vi "TXSIG_Generate(SubVi).vi"(5 "Chip_rate_Threshold":dbl=5.0 format="%#_13g", 7 "ThresHold":dbl=5.0 format="%#_13g", 9 "Rc":dbl=5500.0 format="%#_13g", 10 "길이":i32=256, 11 "이름 또는 상대 경로":string) -> (1 "TXN":dbl[](array[numeric]), 2 "TXP":dbl[](array[numeric]), 4 "TXSIG":waveform(dbl)[](graph))   [LabVIEW 2017]
uses:
  <vilib>/Analysis/NI_AALBase.lvlib
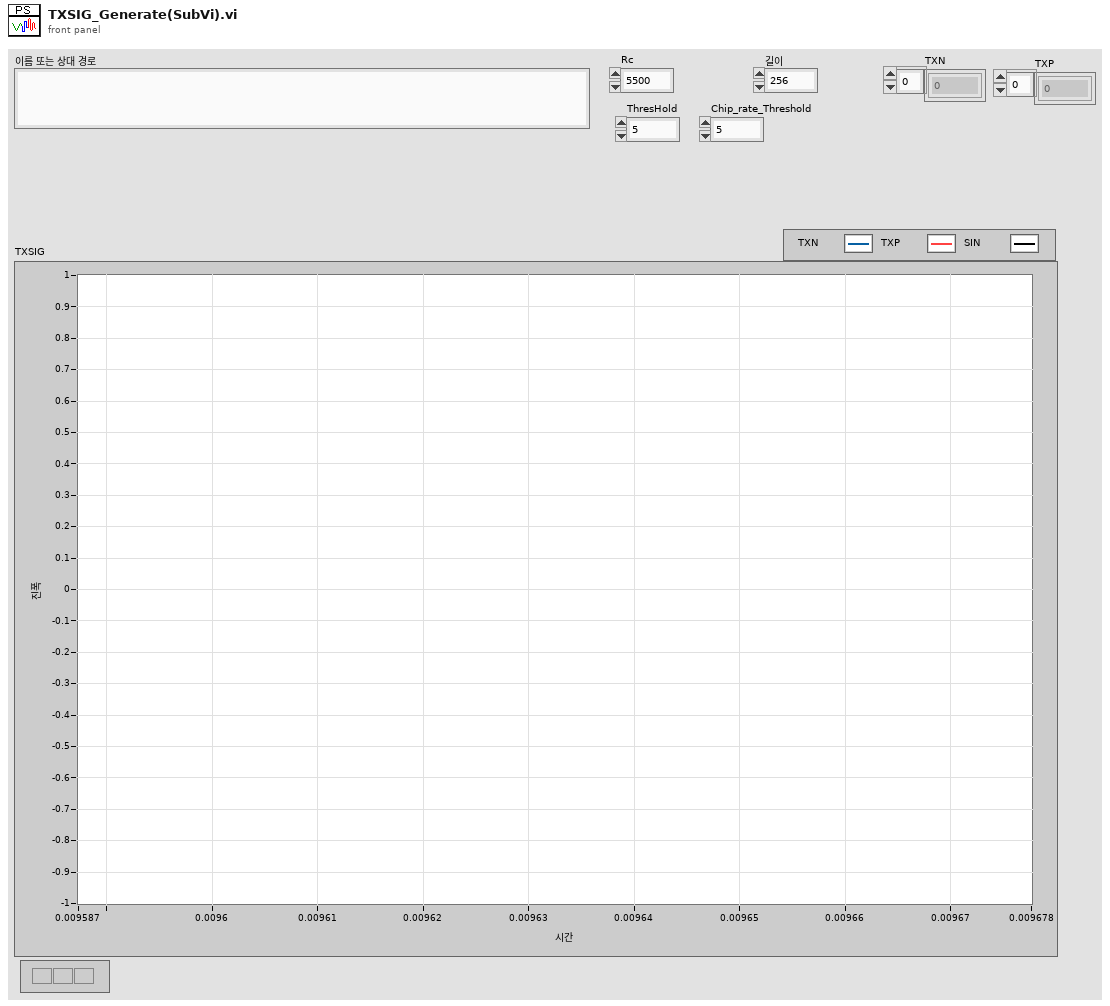
[diagram p1: front panel]
types:
  T1 = enum16{"open", "open or create", "create or replace", "create", "open (read-only)"}
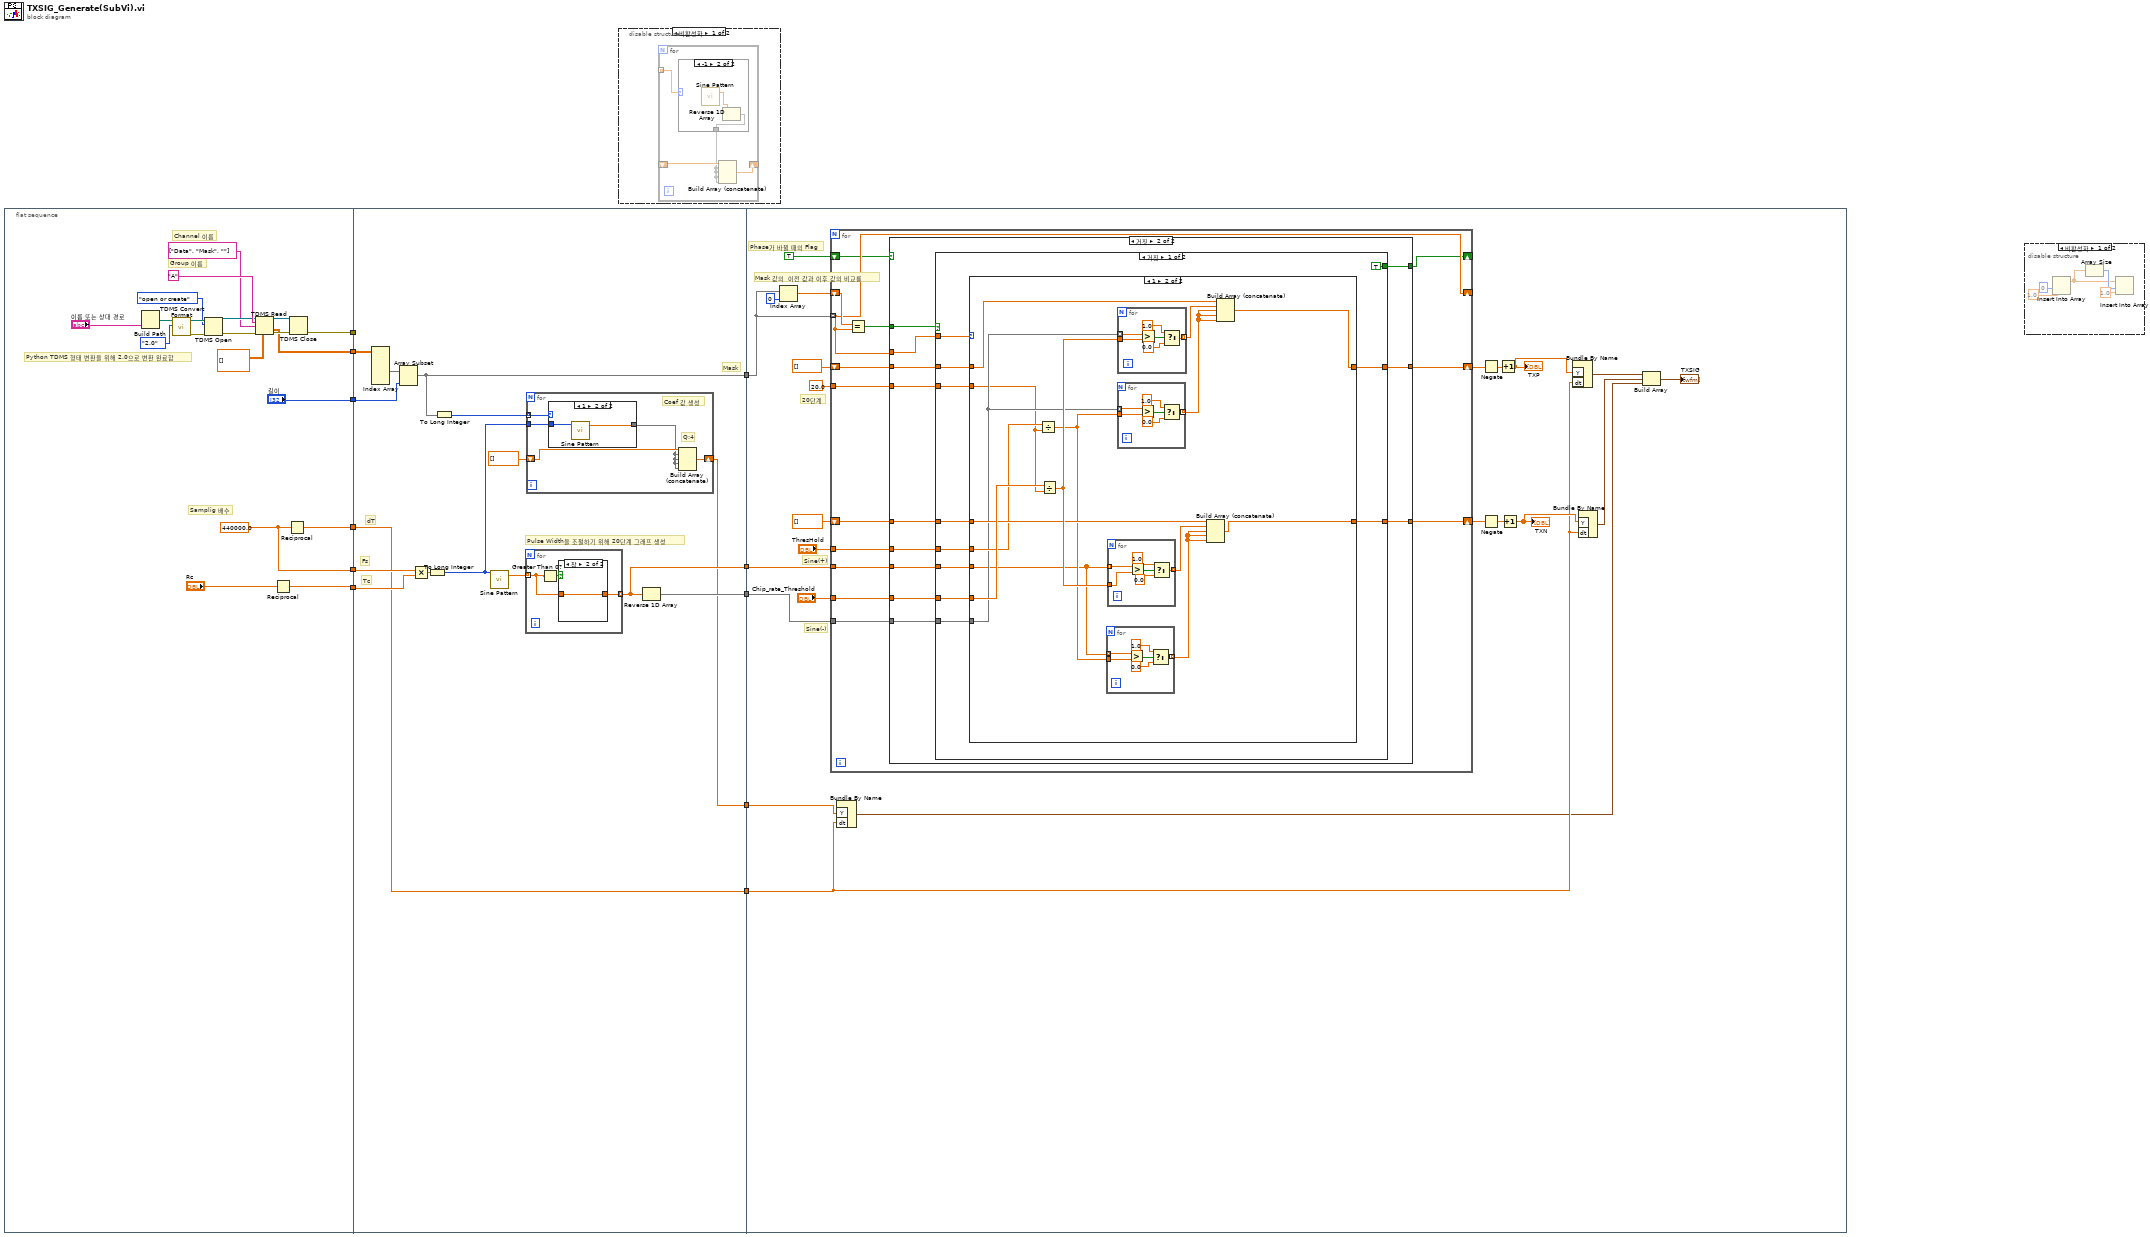
[diagram p0: block diagram]
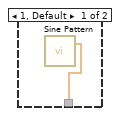
[diagram p2: hidden frame]
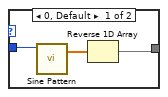
[diagram p5: hidden frame]
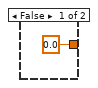
[diagram p6: hidden frame]
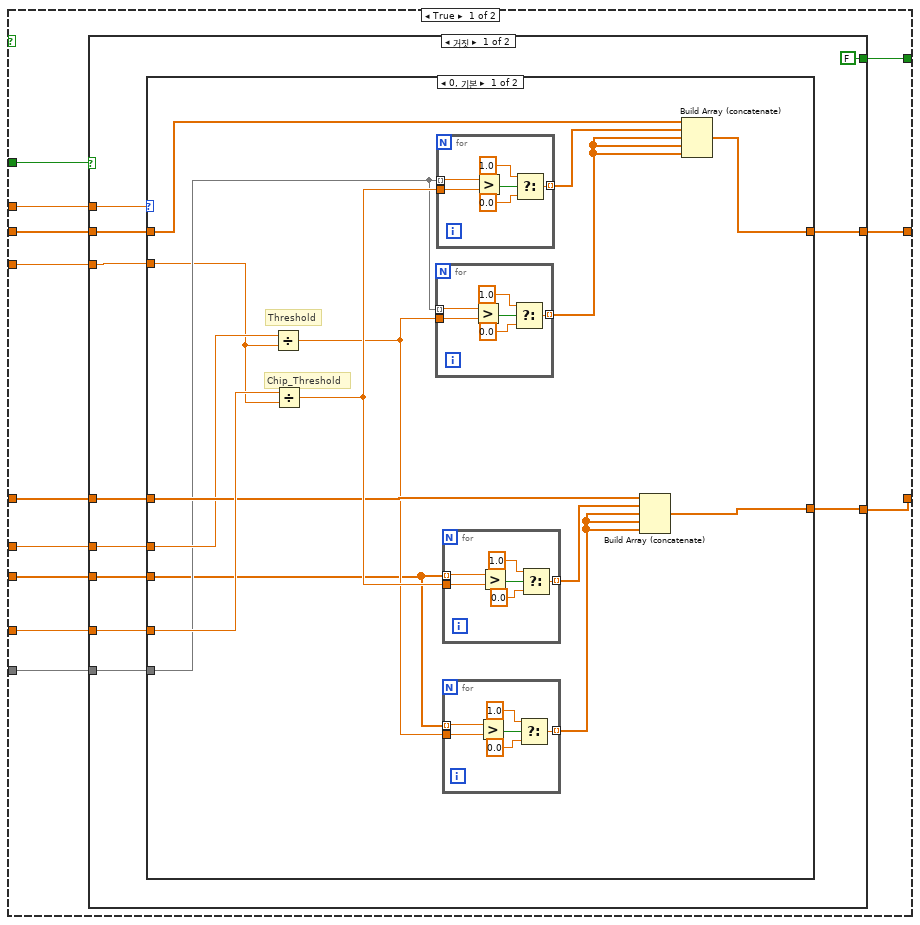
[diagram p7: hidden frame]
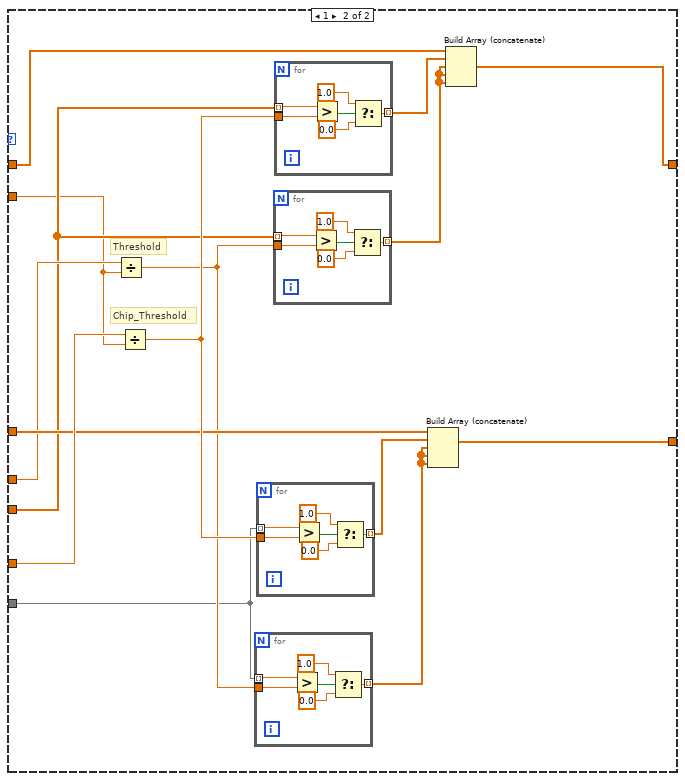
[diagram p8: hidden frame]
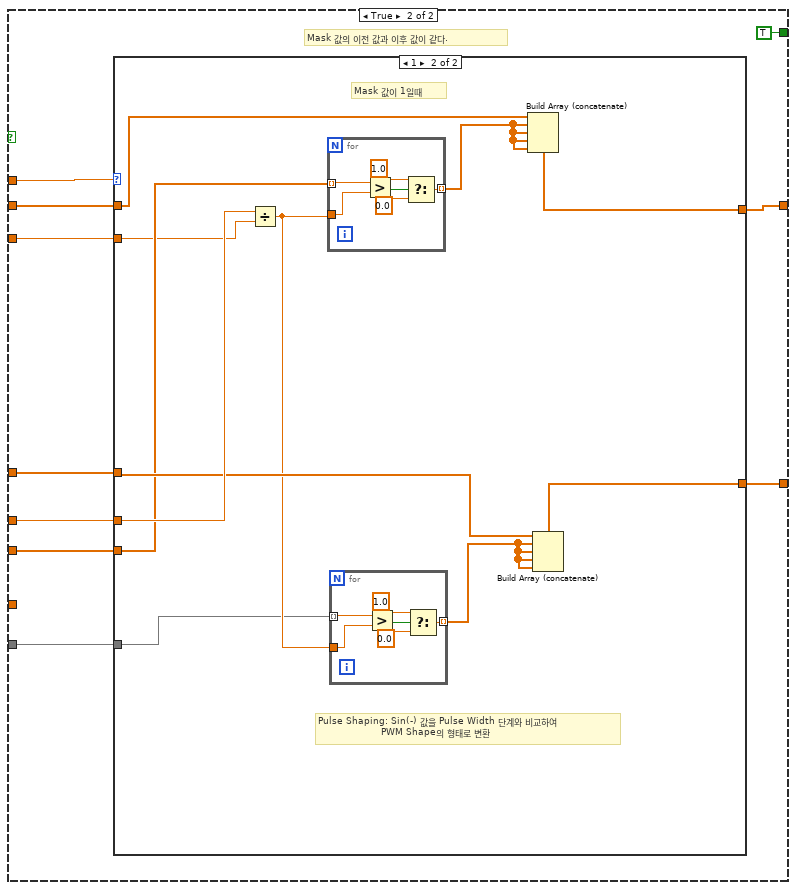
[diagram p9: hidden frame]
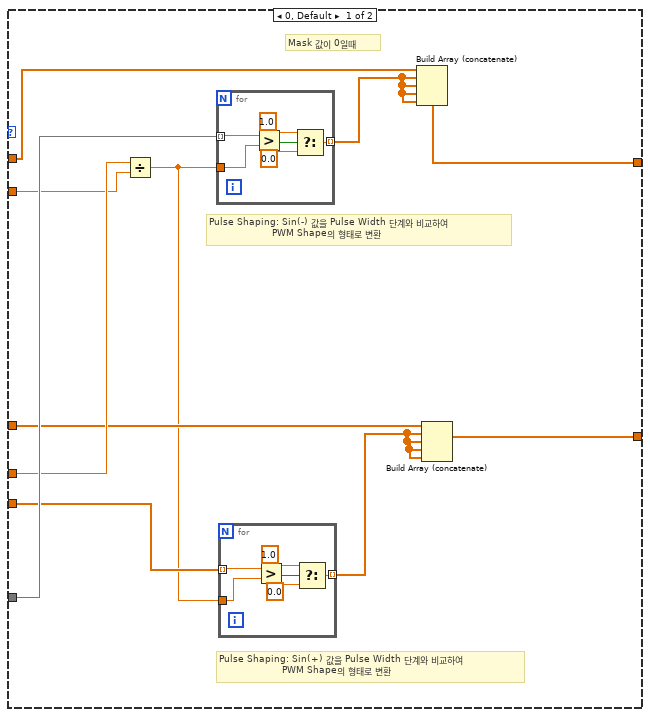
[diagram p10: hidden frame]
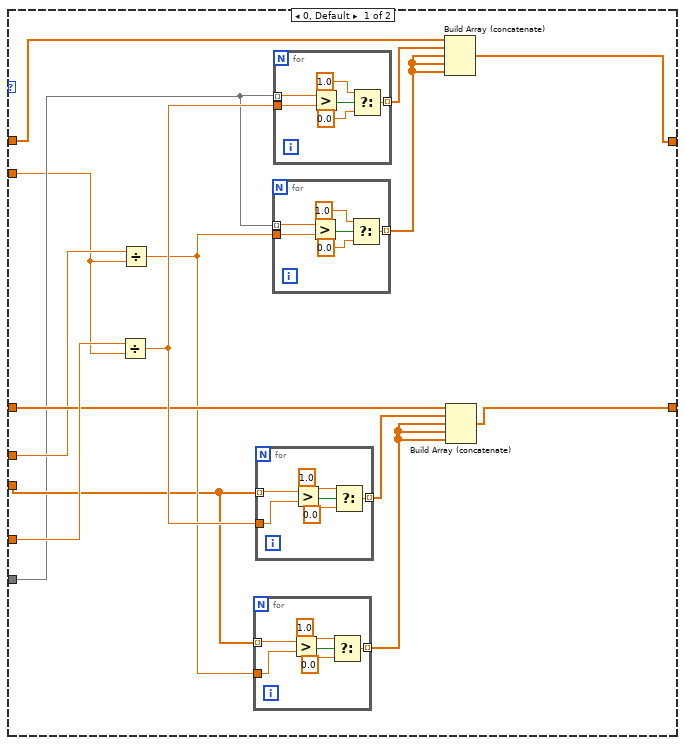
[diagram p11: hidden frame]
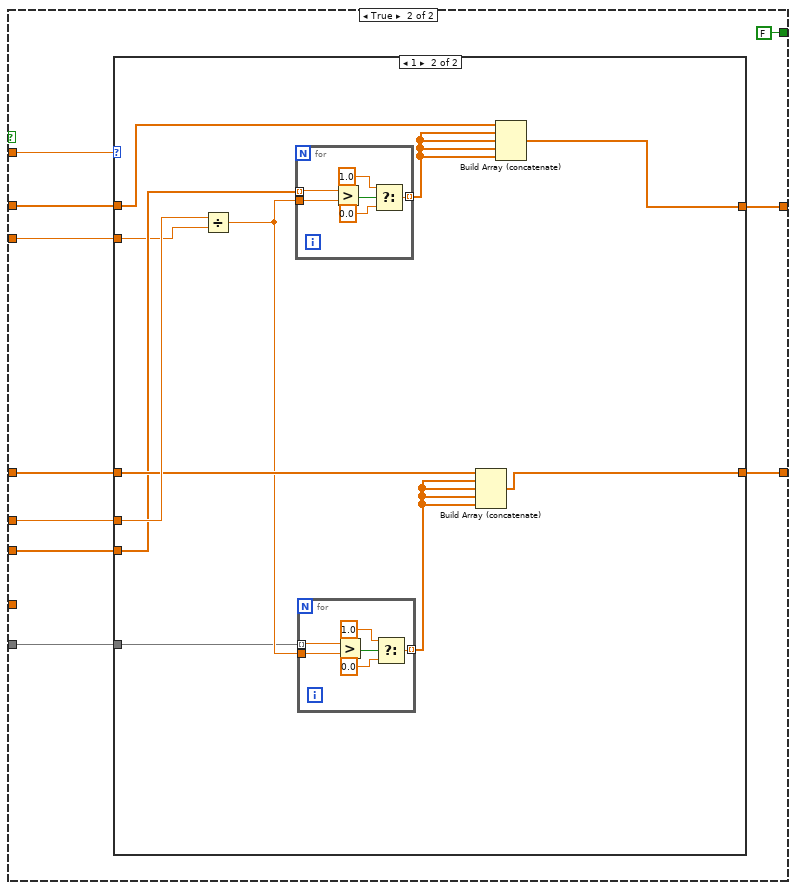
[diagram p12: hidden frame]
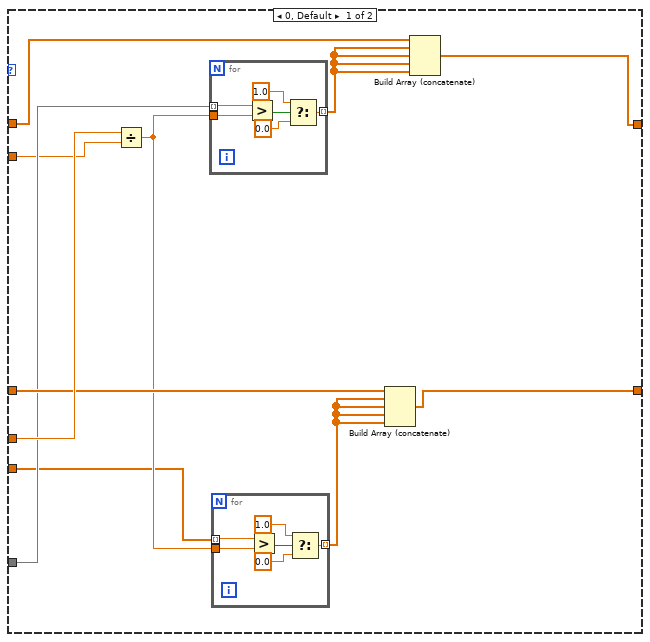
[diagram p13: hidden frame]
diagram:
  n1 = flat-sequence {
    tunnel: [w20] -> w11
    tunnel: [w19] -> w10
    tunnel: ["길이"] -> w6
    tunnel: [w14] -> w5
    tunnel: [w12] -> w4
    tunnel: [w15] -> w3
    tunnel: w10 -> [_]
    tunnel: w11 -> [w43]
    tunnel: [w38] -> w9
    tunnel: [w35] -> w8
    tunnel: [w45] -> w7
    tunnel: w6 -> [w42]
    tunnel: w5 -> [w40]
    tunnel: w4 -> [w39]
    tunnel: w3 -> [w33]
    tunnel: [w34] -> w2
    tunnel: [w33] -> w1
    tunnel: w9 -> [w83]
    tunnel: w8 -> [w80]
    tunnel: w7 -> [w77]
    tunnel: w2 -> [w62]
    tunnel: w1 -> [w67]
    frame #0 {
      w12 = 440000.0
      # "Samplig 배수"
      # "Python TDMS 형태 변환을 위해 2.0으로 변환 완료함"
      # "Group 이름"
      # "Channel 이름"
      n2 = Build Path(name or relative path="이름 또는 상대 경로") -> (appended path=w30:path)  [unwired: 1 in]
      n3 = call <vilib>:"TDMS Convert Format.vi"("target version"=enum16{"1.0", "2.0"}."2.0", "file path"=w30) -> ("error out"=w25:errorcluster, "file path out"=w24:path)  [unwired: 4 in]
      n4 = TDMS Open(8:w25, 10:T1."open or create" ("operation (0:open)"), 11:w24) -> (0:w21:errorcluster, 3:w22:refnum<k34>)  [unwired: 4 in]
      n5 = TDMS Read(0:w22, 5:"A" ("그룹 이름 입력"), 7:string[] ["Data", "Mask", ""] ("채널 이름 입력"), 11:w21, 12:dbl[][] []) -> (4:w27:refnum<k34>, 10:w20:dbl[][], 15:w26:errorcluster)  [unwired: 3 in, 3 out]
      n6 = Reciprocal(x="Rc") -> (1/x=w14:dbl)
      n7 = Reciprocal(x=w12) -> (1/x=w15:dbl)
      n8 = TDMS Close(8:w26, 11:w27) -> (0:w19:errorcluster)  [unwired: 1 out]
    }
    frame #1 {
      # "dT"
      # "Mask"
      # "Pulse Width을 조절하기 위해 20단계 그래프 생성"
      # "Tc"
      # "Fs"
      n9 = Index Array(array=w43) -> (element #2=w44:dbl[])  [unwired: 6 in, 2 out]
      n10 = Array Subset(array=w44, length=w42) -> (w38:dbl[])  [unwired: 1 in]
      n11 = Multiply(x=w39, y=w40) -> (x*y=w41:dbl)
      n12 = To Long Integer(number=w41) -> (32bit integer=w32:i32)
      n13 = To Long Integer(number=w38) -> (32bit integer=w37:i32[])
      n14 = call <vilib>:"Sine Pattern.vi"("samples"=w32) -> ("Sinusoidal Pattern"=w46:dbl[])  [unwired: 3 in, 1 out]
      n15 = for {
        tunnel: w46 -> [w58] mode=indexing
        tunnel: [w57] -> w35 mode=indexing
        n16 = Greater Than 0?(x=w58) -> (x > 0?=w59:bool)
        n17 = case shown="참" w59 {
          tunnel: w58 -> [_ w61]
          tunnel: [0.0 w61] -> w57
          frame False {
          }
          frame True {
          }
        }
      }
      n18 = for {
        tunnel: w32 -> [w51]
        tunnel: w37 -> [w50] mode=indexing
        shift-right: [w47] -> w34
        shift-left: dbl[] [] -> [w49]
        # "Coef 값 생성"
        # "Q:4"
        n19 = case shown="1" w50 {
          tunnel: [w52 w55] -> w48
          tunnel: w51 -> [w54 w56]
          frame 0, Default {
            n20 = call <vilib>:"Sine Pattern.vi"("samples"=w54) -> ("Sinusoidal Pattern"=w53:dbl[])  [unwired: 3 in, 1 out]
            n21 = Reverse 1D Array(array=w53) -> (reversed array=w52:dbl[])
          }
          frame 1 {
            n22 = call <vilib>:"Sine Pattern.vi"("samples"=w56) -> ("Sinusoidal Pattern"=w55:dbl[])  [unwired: 3 in, 1 out]
          }
        }
        n23 = Build Array (concatenate)(w49, w48, w48, w48, w48) -> (w47:dbl[])
      }
      n24 = Reverse 1D Array(array=w35) -> (reversed array=w45:dbl[])
    }
    frame #2 {
      # "20단계"
      # "Mask 값의  이전 값과 이후 값의 비교를"
      # "Phase가 바뀔 때의 Flag"
      # "Sine(-)"
      # "Sine(+)"
      n25 = Index Array(array=w83, index=0 ("인덱스")) -> (element=w81:dbl)
      n26 = for {
        shift-right: [w86] -> _
        shift-left: TRUE -> [w87]
        tunnel: w83 -> [w96] mode=indexing
        shift-right: [w96] -> _
        shift-left: w81 -> [w98]
        tunnel: w80 -> [w95]
        shift-right: [w91] -> w74
        shift-left: dbl[] [] -> [w93]
        shift-right: [w90] -> w73
        shift-left: dbl[] [] -> [w94]
        tunnel: w77 -> [w92]
        tunnel: "ThresHold" -> [w89]
        tunnel: "Chip_rate_Threshold" -> [w88]
        tunnel: 20.0 ("y") -> [w85]
        n27 = Equal?(x=w98, y=w96) -> (x = y?=w97:bool)
        n28 = case shown="거짓" w87 {
          tunnel: w97 -> [w110 w267]
          tunnel: w96 -> [w109 w266]
          tunnel: w95 -> [w108 w265]
          tunnel: w94 -> [w107 w264]
          tunnel: w93 -> [w106 w263]
          tunnel: w92 -> [w105 w262]
          tunnel: [w104 w261] -> w91
          tunnel: [w103 w260] -> w90
          tunnel: w89 -> [w102 w259]
          tunnel: w88 -> [w101 w258]
          tunnel: [w100 w257] -> w86
          tunnel: w85 -> [w99 w256]
          frame True {
            n29 = case shown="거짓" w110 {
              tunnel: w109 -> [w121 w209]
              tunnel: w108 -> [w117 w205]
              tunnel: w107 -> [w119 w208]
              tunnel: w106 -> [w120 w207]
              tunnel: w105 -> [w116 w206]
              tunnel: [w114 w204] -> w104
              tunnel: [w113 w203] -> w103
              tunnel: w102 -> [w118 w202]
              tunnel: w101 -> [w115 _]
              tunnel: [FALSE TRUE] -> w100
              tunnel: w99 -> [w111 w200]
              frame False {
                n30 = case shown="0, 기본" w121 {
                  tunnel: w120 -> [w136 w175]
                  tunnel: w119 -> [w132 w171]
                  tunnel: w118 -> [w128 w167]
                  tunnel: w117 -> [w124 w163]
                  tunnel: w116 -> [w127 w162]
                  tunnel: w115 -> [w135 w174]
                  tunnel: [w134 w173] -> w114
                  tunnel: [w131 w170] -> w113
                  tunnel: w111 -> [w122 w161]
                  frame 0, Default {
                    # "Threshold"
                    # "Chip_Threshold"
                    n31 = Divide(x=w128, y=w122) -> (x/y=w125:dbl)
                    n32 = Divide(x=w135, y=w122) -> (x/y=w133:dbl)
                    n33 = for {
                      tunnel: w127 -> [w148] mode=indexing
                      tunnel: w125 -> [w147]
                      tunnel: [w143] -> w126 mode=indexing
                      n34 = Greater?(x=w148, y=w147) -> (0:w146:bool)
                      n35 = Select(t=1.0, s=w146, f=0.0) -> (s? t:f=w143:dbl)
                    }
                    n36 = for {
                      tunnel: w127 -> [w160] mode=indexing
                      tunnel: w133 -> [w159]
                      tunnel: [w155] -> w130 mode=indexing
                      n37 = Greater?(x=w160, y=w159) -> (0:w158:bool)
                      n38 = Select(t=1.0, s=w158, f=0.0) -> (s? t:f=w155:dbl)
                    }
                    n39 = for {
                      tunnel: w124 -> [w154] mode=indexing
                      tunnel: w133 -> [w153]
                      tunnel: [w149] -> w129 mode=indexing
                      n40 = Greater?(x=w154, y=w153) -> (0:w152:bool)
                      n41 = Select(t=1.0, s=w152, f=0.0) -> (s? t:f=w149:dbl)
                    }
                    n42 = for {
                      tunnel: w124 -> [w142] mode=indexing
                      tunnel: w125 -> [w141]
                      tunnel: [w137] -> w123 mode=indexing
                      n43 = Greater?(x=w142, y=w141) -> (0:w140:bool)
                      n44 = Select(t=1.0, s=w140, f=0.0) -> (s? t:f=w137:dbl)
                    }
                    n45 = Build Array (concatenate)(w132, w129, w123, w123, w123) -> (w131:dbl[])
                    n46 = Build Array (concatenate)(w136, w130, w126, w126, w126) -> (w134:dbl[])
                  }
                  frame 1 {
                    # "Chip_Threshold"
                    # "Threshold"
                    n47 = Divide(x=w167, y=w161) -> (x/y=w165:dbl)
                    n48 = Divide(x=w174, y=w161) -> (x/y=w172:dbl)
                    n49 = for {
                      tunnel: w162 -> [w181] mode=indexing
                      tunnel: w165 -> [w180]
                      tunnel: [w176] -> w164 mode=indexing
                      n50 = Greater?(x=w181, y=w180) -> (0:w179:bool)
                      n51 = Select(t=1.0, s=w179, f=0.0) -> (s? t:f=w176:dbl)
                    }
                    n52 = for {
                      tunnel: w162 -> [w193] mode=indexing
                      tunnel: w172 -> [w192]
                      tunnel: [w188] -> w168 mode=indexing
                      n53 = Greater?(x=w193, y=w192) -> (0:w191:bool)
                      n54 = Select(t=1.0, s=w191, f=0.0) -> (s? t:f=w188:dbl)
                    }
                    n55 = for {
                      tunnel: w163 -> [w187] mode=indexing
                      tunnel: w165 -> [w186]
                      tunnel: [w182] -> w166 mode=indexing
                      n56 = Greater?(x=w187, y=w186) -> (0:w185:bool)
                      n57 = Select(t=1.0, s=w185, f=0.0) -> (s? t:f=w182:dbl)
                    }
                    n58 = for {
                      tunnel: w163 -> [w199] mode=indexing
                      tunnel: w172 -> [w198]
                      tunnel: [w194] -> w169 mode=indexing
                      n59 = Greater?(x=w199, y=w198) -> (0:w197:bool)
                      n60 = Select(t=1.0, s=w197, f=0.0) -> (s? t:f=w194:dbl)
                    }
                    n61 = Build Array (concatenate)(w171, w168, w164, w164, w164) -> (w170:dbl[])
                    n62 = Build Array (concatenate)(w175, w169, w166, w166, w166) -> (w173:dbl[])
                  }
                }
              }
              frame True {
                # "Mask 값의 이전 값과 이후 값이 같다."
                n63 = case shown="1" w209 {
                  tunnel: w208 -> [w216 w240]
                  tunnel: w207 -> [w220 w243]
                  tunnel: w206 -> [w218 w235]
                  tunnel: w205 -> [w215 w234]
                  tunnel: [w219 w242] -> w204
                  tunnel: [w213 w238] -> w203
                  tunnel: w202 -> [w217 w241]
                  tunnel: w200 -> [w210 w233]
                  frame 0, Default {
                    # "Pulse Shaping: Sin(+) 값을 Pulse Width 단계와 비교하여\n                     PWM Shape의 형태로 변환"
                    # "Pulse Shaping: Sin(-) 값을 Pulse Width 단계와 비교하여\n                     PWM Shape의 형태로 변환"
                    # "Mask 값이 0일때"
                    n64 = Divide(x=w217, y=w210) -> (x/y=w214:dbl)
                    n65 = for {
                      tunnel: w218 -> [w232] mode=indexing
                      tunnel: w214 -> [w231]
                      tunnel: [w227] -> w212 mode=indexing
                      n66 = Greater?(x=w232, y=w231) -> (0:w230:bool)
                      n67 = Select(t=1.0, s=w230, f=0.0) -> (s? t:f=w227:dbl)
                    }
                    n68 = for {
                      tunnel: w215 -> [w226] mode=indexing
                      tunnel: w214 -> [w225]
                      tunnel: [w221] -> w211 mode=indexing
                      n69 = Greater?(x=w226, y=w225) -> (0:w224:bool)
                      n70 = Select(t=1.0, s=w224, f=0.0) -> (s? t:f=w221:dbl)
                    }
                    n71 = Build Array (concatenate)(w220, w212, w212, w212, w212) -> (w219:dbl[])
                    n72 = Build Array (concatenate)(w216, w211, w211, w211, w211) -> (w213:dbl[])
                  }
                  frame 1 {
                    # "Pulse Shaping: Sin(-) 값을 Pulse Width 단계와 비교하여\n                     PWM Shape의 형태로 변환"
                    # "Mask 값이 1일때"
                    n73 = Divide(x=w241, y=w233) -> (x/y=w239:dbl)
                    n74 = for {
                      tunnel: w234 -> [w255] mode=indexing
                      tunnel: w239 -> [w254]
                      tunnel: [w250] -> w237 mode=indexing
                      n75 = Greater?(x=w255, y=w254) -> (0:w253:bool)
                      n76 = Select(t=1.0, s=w253, f=0.0) -> (s? t:f=w250:dbl)
                    }
                    n77 = for {
                      tunnel: w235 -> [w249] mode=indexing
                      tunnel: w239 -> [w248]
                      tunnel: [w244] -> w236 mode=indexing
                      n78 = Greater?(x=w249, y=w248) -> (0:w247:bool)
                      n79 = Select(t=1.0, s=w247, f=0.0) -> (s? t:f=w244:dbl)
                    }
                    n80 = Build Array (concatenate)(w243, w237, w237, w237, w237) -> (w242:dbl[])
                    n81 = Build Array (concatenate)(w240, w236, w236, w236, w236) -> (w238:dbl[])
                  }
                }
              }
            }
          }
          frame False {
            n82 = case shown="거짓" w267 {
              tunnel: w266 -> [w278 w366]
              tunnel: w265 -> [w274 w362]
              tunnel: w264 -> [w276 w365]
              tunnel: w263 -> [w277 w364]
              tunnel: w262 -> [w273 w363]
              tunnel: [w271 w361] -> w261
              tunnel: [w270 w360] -> w260
              tunnel: w259 -> [w275 w359]
              tunnel: w258 -> [w272 _]
              tunnel: [TRUE FALSE] -> w257
              tunnel: w256 -> [w268 w357]
              frame False {
                n83 = case shown="1" w278 {
                  tunnel: w277 -> [w293 w332]
                  tunnel: w276 -> [w289 w328]
                  tunnel: w275 -> [w285 w324]
                  tunnel: w274 -> [w282 w319]
                  tunnel: w273 -> [w281 w320]
                  tunnel: w272 -> [w292 w331]
                  tunnel: [w291 w330] -> w271
                  tunnel: [w288 w327] -> w270
                  tunnel: w268 -> [w280 w318]
                  frame 0, Default {
                    n84 = Divide(x=w292, y=w280) -> (x/y=w290:dbl)
                    n85 = Divide(x=w285, y=w280) -> (x/y=w283:dbl)
                    n86 = for {
                      tunnel: w282 -> [w299] mode=indexing
                      tunnel: w283 -> [w298]
                      tunnel: [w294] -> w279 mode=indexing
                      n87 = Greater?(x=w299, y=w298) -> (0:w297:bool)
                      n88 = Select(t=1.0, s=w297, f=0.0) -> (s? t:f=w294:dbl)
                    }
                    n89 = for {
                      tunnel: w282 -> [w311] mode=indexing
                      tunnel: w290 -> [w310]
                      tunnel: [w306] -> w286 mode=indexing
                      n90 = Greater?(x=w311, y=w310) -> (0:w309:bool)
                      n91 = Select(t=1.0, s=w309, f=0.0) -> (s? t:f=w306:dbl)
                    }
                    n92 = for {
                      tunnel: w281 -> [w305] mode=indexing
                      tunnel: w283 -> [w304]
                      tunnel: [w300] -> w284 mode=indexing
                      n93 = Greater?(x=w305, y=w304) -> (0:w303:bool)
                      n94 = Select(t=1.0, s=w303, f=0.0) -> (s? t:f=w300:dbl)
                    }
                    n95 = for {
                      tunnel: w281 -> [w317] mode=indexing
                      tunnel: w290 -> [w316]
                      tunnel: [w312] -> w287 mode=indexing
                      n96 = Greater?(x=w317, y=w316) -> (0:w315:bool)
                      n97 = Select(t=1.0, s=w315, f=0.0) -> (s? t:f=w312:dbl)
                    }
                    n98 = Build Array (concatenate)(w293, w287, w284, w284, w284) -> (w291:dbl[])
                    n99 = Build Array (concatenate)(w289, w286, w279, w279, w279) -> (w288:dbl[])
                  }
                  frame 1 {
                    n100 = Divide(x=w324, y=w318) -> (x/y=w322:dbl)
                    n101 = Divide(x=w331, y=w318) -> (x/y=w329:dbl)
                    n102 = for {
                      tunnel: w319 -> [w338] mode=indexing
                      tunnel: w322 -> [w337]
                      tunnel: [w333] -> w321 mode=indexing
                      n103 = Greater?(x=w338, y=w337) -> (0:w336:bool)
                      n104 = Select(t=1.0, s=w336, f=0.0) -> (s? t:f=w333:dbl)
                    }
                    n105 = for {
                      tunnel: w319 -> [w350] mode=indexing
                      tunnel: w329 -> [w349]
                      tunnel: [w345] -> w325 mode=indexing
                      n106 = Greater?(x=w350, y=w349) -> (0:w348:bool)
                      n107 = Select(t=1.0, s=w348, f=0.0) -> (s? t:f=w345:dbl)
                    }
                    n108 = for {
                      tunnel: w320 -> [w344] mode=indexing
                      tunnel: w322 -> [w343]
                      tunnel: [w339] -> w323 mode=indexing
                      n109 = Greater?(x=w344, y=w343) -> (0:w342:bool)
                      n110 = Select(t=1.0, s=w342, f=0.0) -> (s? t:f=w339:dbl)
                    }
                    n111 = for {
                      tunnel: w320 -> [w356] mode=indexing
                      tunnel: w329 -> [w355]
                      tunnel: [w351] -> w326 mode=indexing
                      n112 = Greater?(x=w356, y=w355) -> (0:w354:bool)
                      n113 = Select(t=1.0, s=w354, f=0.0) -> (s? t:f=w351:dbl)
                    }
                    n114 = Build Array (concatenate)(w328, w325, w321, w321, w321) -> (w327:dbl[])
                    n115 = Build Array (concatenate)(w332, w326, w323, w323, w323) -> (w330:dbl[])
                  }
                }
              }
              frame True {
                n116 = case shown="1" w366 {
                  tunnel: w365 -> [w374 w397]
                  tunnel: w364 -> [w377 w400]
                  tunnel: w363 -> [w369 w392]
                  tunnel: w362 -> [w368 w391]
                  tunnel: [w376 w399] -> w361
                  tunnel: [w372 w395] -> w360
                  tunnel: w359 -> [w375 w398]
                  tunnel: w357 -> [w367 w390]
                  frame 0, Default {
                    n117 = Divide(x=w375, y=w367) -> (x/y=w373:dbl)
                    n118 = for {
                      tunnel: w369 -> [w389] mode=indexing
                      tunnel: w373 -> [w388]
                      tunnel: [w384] -> w371 mode=indexing
                      n119 = Greater?(x=w389, y=w388) -> (0:w387:bool)
                      n120 = Select(t=1.0, s=w387, f=0.0) -> (s? t:f=w384:dbl)
                    }
                    n121 = for {
                      tunnel: w368 -> [w383] mode=indexing
                      tunnel: w373 -> [w382]
                      tunnel: [w378] -> w370 mode=indexing
                      n122 = Greater?(x=w383, y=w382) -> (0:w381:bool)
                      n123 = Select(t=1.0, s=w381, f=0.0) -> (s? t:f=w378:dbl)
                    }
                    n124 = Build Array (concatenate)(w374, w370, w370, w370, w370) -> (w372:dbl[])
                    n125 = Build Array (concatenate)(w377, w371, w371, w371, w371) -> (w376:dbl[])
                  }
                  frame 1 {
                    n126 = Divide(x=w398, y=w390) -> (x/y=w396:dbl)
                    n127 = for {
                      tunnel: w391 -> [w412] mode=indexing
                      tunnel: w396 -> [w411]
                      tunnel: [w407] -> w394 mode=indexing
                      n128 = Greater?(x=w412, y=w411) -> (0:w410:bool)
                      n129 = Select(t=1.0, s=w410, f=0.0) -> (s? t:f=w407:dbl)
                    }
                    n130 = for {
                      tunnel: w392 -> [w406] mode=indexing
                      tunnel: w396 -> [w405]
                      tunnel: [w401] -> w393 mode=indexing
                      n131 = Greater?(x=w406, y=w405) -> (0:w404:bool)
                      n132 = Select(t=1.0, s=w404, f=0.0) -> (s? t:f=w401:dbl)
                    }
                    n133 = Build Array (concatenate)(w397, w393, w393, w393, w393) -> (w395:dbl[])
                    n134 = Build Array (concatenate)(w400, w394, w394, w394, w394) -> (w399:dbl[])
                  }
                }
              }
            }
          }
        }
      }
      n135 = Bundle By Name("Y"=w62, "dt"=w67) -> (w64:waveform(dbl))  [unwired: 1 in]
      n136 = Negate(x=w74) -> (-x=w72:dbl[])
      n137 = Negate(x=w73) -> (-x=w71:dbl[])
      n138 = Increment(x=w72) -> (x+1=w69:dbl[])
      "TXP" <- w69
      n139 = Increment(x=w71) -> (x+1=w68:dbl[])
      "TXN" <- w68
      n140 = Bundle By Name("Y"=w69, "dt"=w67) -> (w66:waveform(dbl))  [unwired: 1 in]
      n141 = Bundle By Name("Y"=w68, "dt"=w67) -> (w65:waveform(dbl))  [unwired: 1 in]
      n142 = Build Array(w66, w65, w64) -> (→"TXSIG":waveform(dbl)[])
    }
  }
  n143 = disable-structure shown="비활성화" {
    frame Disabled {
      n144 = for {
        tunnel: _ -> [w416] mode=indexing
        shift-right: [w414] -> _
        shift-left: _ -> [w415]
        n145 = case shown="-1" w416 {
          tunnel: [w417 w418] -> w413
          frame 1, Default {
            n146 = call <vilib>:"Sine Pattern.vi"() -> ("Sinusoidal Pattern"=w417:dbl[])  [unwired: 4 in, 1 out]
          }
          frame -1 {
            n147 = call <vilib>:"Sine Pattern.vi"() -> ("Sinusoidal Pattern"=w419:dbl[])  [unwired: 4 in, 1 out]
            n148 = Reverse 1D Array(array=w419) -> (reversed array=w418:dbl[])
          }
        }
        n149 = Build Array (concatenate)(w415, w413, w413, w413, w413) -> (w414:dbl[])
      }
    }
    frame Enabled {
    }
  }
  n150 = disable-structure shown="비활성화" {
    frame Disabled {
      n151 = Insert Into Array(index=0 ("인덱스"), new element=1.0 ("새 원소/부분배열")) -> (w422:dbl[])  [unwired: 1 in]
      n152 = Array Size(array=w422) -> (size(s)=w423:i32)
      n153 = Insert Into Array(array=w422, index=w423, new element=1.0 ("새 원소/부분배열")) -> ()  [unwired: 1 out]
    }
    frame Enabled {
    }
  }
